vi "StatsTVE.vi"(8 "error in (no error)":errorcluster, 11 "ResultArrayIn":T1 {"Time Stamp" format="%^<%.3X\n%x>T"}) -> (0 "error out":errorcluster, 1 "StringArray":string[][](array[string]), 2 "StatArray":dbl[][](array[numeric]), 3 "ResultArrayOut":T1 {"Time Stamp" format="%^<%.3X\n%x>T"})   [LabVIEW 2014]
uses:
  typedefs/ResultArray.ctl
  typedefs/Result.ctl
  typedefs/TVE_Fe_RFE.ctl
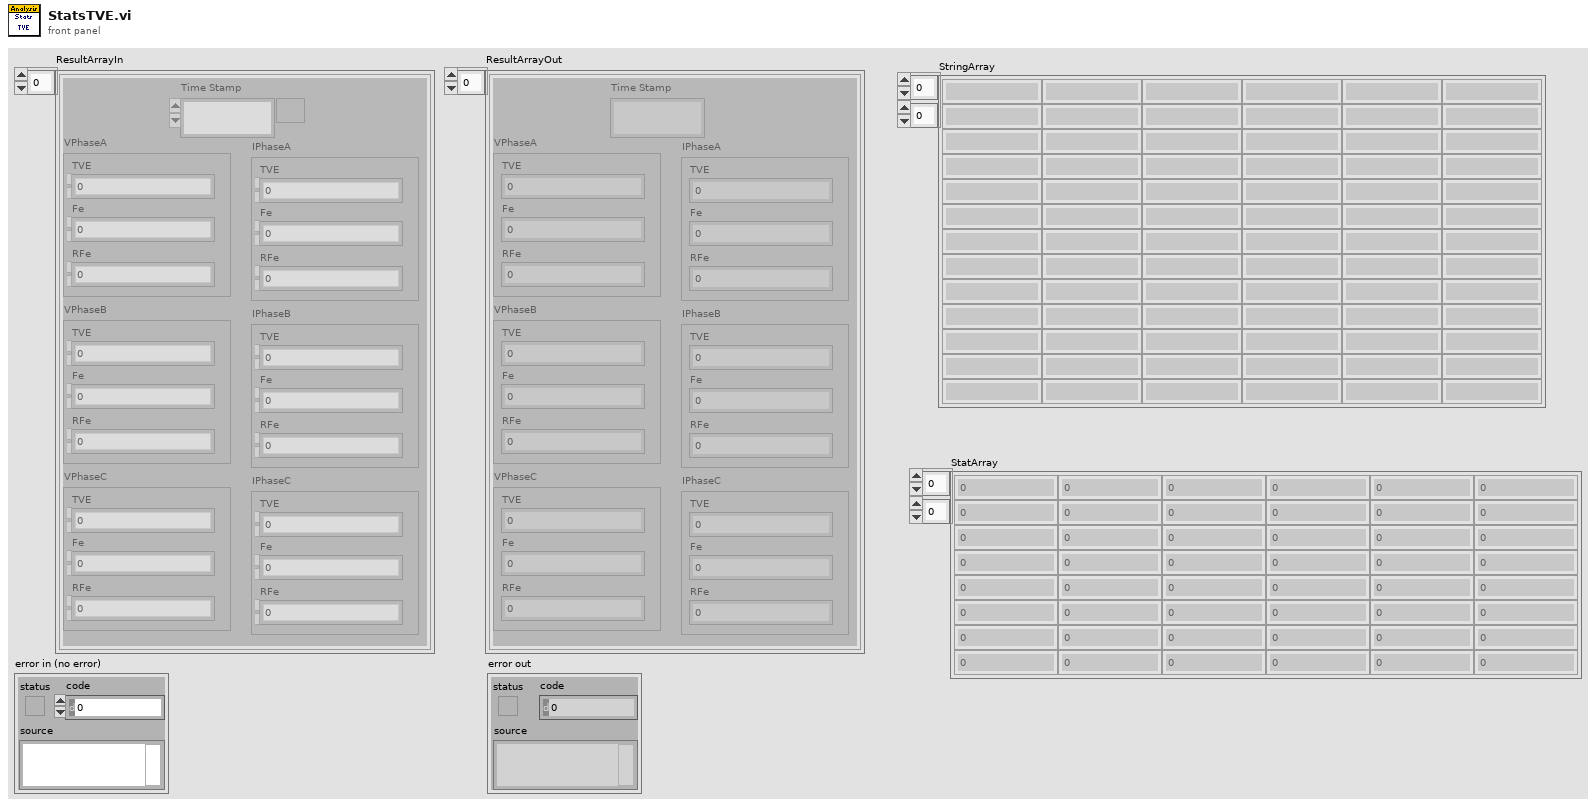
[diagram p1: front panel]
types:
  T1 = typedef "ResultArray.ctl" = T2[]
  T2 = typedef "Result.ctl" = cluster{"Time Stamp":timestamp, "VPhaseA":T3, "VPhaseB":T3, "VPhaseC":T3, "IPhaseA":T3, "IPhaseB":T3, "IPhaseC":T3}
  T3 = typedef "TVE_Fe_RFE.ctl" = cluster{"TVE":dbl, "Fe":dbl, "RFe":dbl}
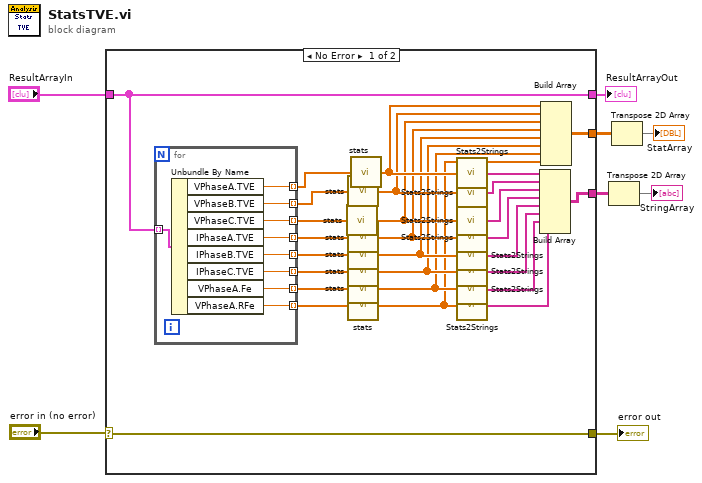
[diagram p0: block diagram]
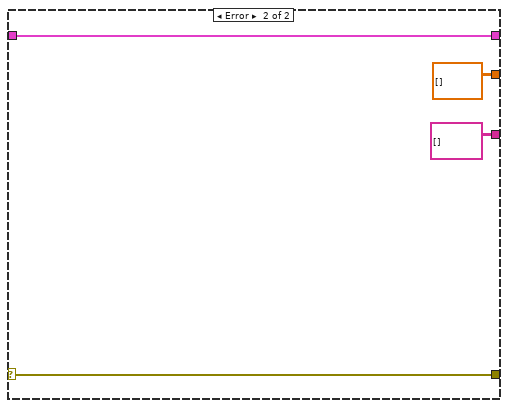
[diagram p2: hidden frame]
diagram:
  n1 = case shown="No Error" "error in (no error)" {
    selector: "error in (no error)" -> [w15 w48]
    tunnel: "ResultArrayIn" -> [w36 w49]
    tunnel: [w36 w49] -> w6
    tunnel: [w15 w48] -> w5
    tunnel: [w17 dbl[][] []] -> w4
    tunnel: [w16 string[][] []] -> w3
    frame No Error {
      n2 = for {
        tunnel: w36 -> [w45] mode=indexing
        tunnel: [w44] -> w35 mode=indexing
        tunnel: [w43] -> w34 mode=indexing
        tunnel: [w42] -> w33 mode=indexing
        tunnel: [w41] -> w32 mode=indexing
        tunnel: [w40] -> w31 mode=indexing
        tunnel: [w39] -> w30 mode=indexing
        tunnel: [w38] -> w14 mode=indexing
        tunnel: [w37] -> w13 mode=indexing
        n3 = Unbundle By Name(w45) -> ("VPhaseA.TVE"=w44:dbl, "VPhaseB.TVE"=w43:dbl, "VPhaseC.TVE"=w42:dbl, "IPhaseA.TVE"=w41:dbl, "IPhaseB.TVE"=w40:dbl, "IPhaseC.TVE"=w39:dbl, "VPhaseA.Fe"=w38:dbl, "VPhaseA.RFe"=w37:dbl)
      }
      n4 = call "stats.vi"("ArrayIn"=w33) -> ("stats"=w26:dbl[])  [unwired: 8 in]
      n5 = call "stats.vi"("ArrayIn"=w34) -> ("stats"=w27:dbl[])  [unwired: 8 in]
      n6 = call "stats.vi"("ArrayIn"=w32) -> ("stats"=w25:dbl[])  [unwired: 8 in]
      n7 = call "stats.vi"("ArrayIn"=w31) -> ("stats"=w24:dbl[])  [unwired: 8 in]
      n8 = call "stats.vi"("ArrayIn"=w30) -> ("stats"=w23:dbl[])  [unwired: 8 in]
      n9 = call "stats.vi"("ArrayIn"=w14) -> ("stats"=w12:dbl[])  [unwired: 8 in]
      n10 = call "stats.vi"("ArrayIn"=w13) -> ("stats"=w11:dbl[])  [unwired: 8 in]
      n11 = call "stats.vi"("ArrayIn"=w35) -> ("stats"=w29:dbl[])  [unwired: 8 in]
      n12 = call "Stats2Strings.vi"("stats"=w29) -> ("Strings"=w28:string[])  [unwired: 8 in]
      n13 = call "Stats2Strings.vi"("stats"=w27) -> ("Strings"=w22:string[])  [unwired: 8 in]
      n14 = call "Stats2Strings.vi"("stats"=w26) -> ("Strings"=w21:string[])  [unwired: 8 in]
      n15 = call "Stats2Strings.vi"("stats"=w25) -> ("Strings"=w20:string[])  [unwired: 8 in]
      n16 = call "Stats2Strings.vi"("stats"=w24) -> ("Strings"=w19:string[])  [unwired: 8 in]
      n17 = call "Stats2Strings.vi"("stats"=w23) -> ("Strings"=w18:string[])  [unwired: 8 in]
      n18 = call "Stats2Strings.vi"("stats"=w12) -> ("Strings"=w10:string[])  [unwired: 8 in]
      n19 = call "Stats2Strings.vi"("stats"=w11) -> ("Strings"=w9:string[])  [unwired: 8 in]
      n20 = Build Array(w28, w22, w21, w20, w19, w18, w10, w9) -> (w16:string[][])
      n21 = Build Array(w29, w27, w26, w25, w24, w23, w12, w11) -> (w17:dbl[][])
    }
    frame Error {
    }
  }
  "ResultArrayOut" <- w6
  "error out" <- w5
  n22 = Transpose 2D Array(2D array=w3) -> (transposed array=→"StringArray":string[][])
  n23 = Transpose 2D Array(2D array=w4) -> (transposed array=→"StatArray":dbl[][])
